vi "format set align.vi"(8 "error in (no error)":errorcluster, 10 "alignment":T1 items=["LXW_ALIGN_NONE", "LXW_ALIGN_LEFT", "LXW_ALIGN_CENTER", "LXW_ALIGN_RIGHT", "LXW_ALIGN_FILL", "LXW_ALIGN_JUSTIFY", "LXW_ALIGN_CENTER_ACROSS", "LXW_ALIGN_DISTRIBUTED", "LXW_ALIGN_VERTICAL_TOP", "LXW_ALIGN_VERTICAL_BOTTOM", "LXW_ALIGN_VERTICAL_CENTER", "LXW_ALIGN_VERTICAL_JUSTIFY", "LXW_ALIGN_VERTICAL_DISTRIBUTED"], 11 "format":u32) -> (0 "error out":errorcluster)   [LabVIEW 2015, in "xlsxwriter.lvlib"]
doc: "void format_set_align(lxw_format format, uint8_t alignment);"
uses:
  xlsxwriter.lvlib
  Controls/lxw_alignment.ctl
  xlsxwriter.dll
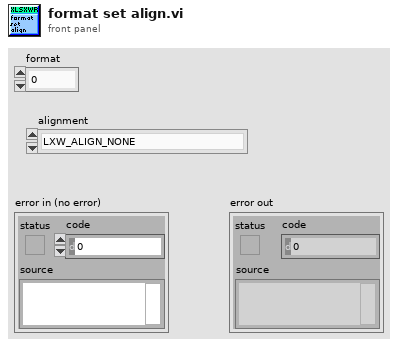
[diagram p1: front panel]
types:
  T1 = typedef "lxw_alignment.ctl" = u8
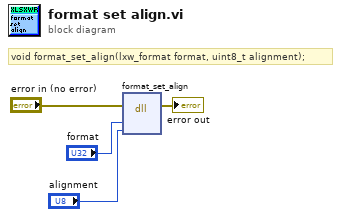
[diagram p0: block diagram]
diagram:
  # "void format_set_align(lxw_format format, uint8_t alignment);"
  n1 = dll-call lib="C:/Users/WDAGUtilityAccount/Desktop/Labview_Example-win32/xlsxwriter.*" fn="format_set_align"(error in="error in (no error)", "format"="format", "alignment"="alignment") -> (error out=→"error out":errorcluster)  [unwired: 5 in, 1 out]
